vi "GetValues.vi"(2 "String":string) -> (6 "Values":u64[](array[numeric]))   [LabVIEW 2022 SP3]
uses:
  <vilib>/regexp/Match Regular Expression.xnode
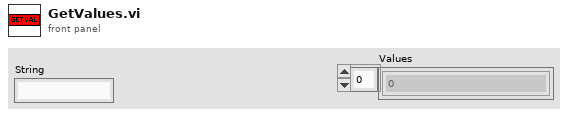
[diagram p1: front panel]
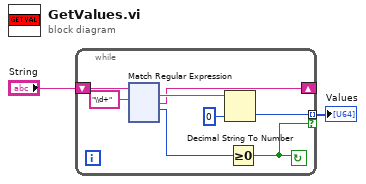
[diagram p0: block diagram]
diagram:
  n1 = while {
    tunnel: [w4] -> w1 mode=indexing if=w5
    shift-right: [w7] -> _
    shift-left: "String" -> [w10]
    stop <- w5 continue-if-true
    n2 = xnode "Match Regular Expression"("input string"=w10, "regular expression"="\\d+") -> ("whole match"=w8:string, "after match"=w7:string, "offset past match"=w6:i32)  [unwired: 4 in, 2 out]
    n3 = Decimal String To Number(string=w8, default (0L)=u64 0 ("default (0 I32)")) -> (number=w4:u64)  [unwired: 1 in, 1 out]
    n4 = Greater Or Equal To 0?(x=w6) -> (x >= 0?=w5:bool)
  }
  "Values" <- w1
